vi "GetConnectorPaneTemplateForExecutionMode.vi"(8 "error in (no error)":errorcluster, 11 "execution mode":T2) -> (0 "error out":errorcluster, 3 "connector pane template":T1)   [LabVIEW 2015, in "VeriStandTestUtilities.lvlib"]
uses:
  VeriStandTestUtilities.lvlib
  <vilib>/NI Veristand/Custom Device API/Custom Device Execution Mode.ctl
  ConnectorPaneTemplate.ctl
  <userlib>/_OpenG.lib/file/file.llb/Build Path - Traditional - path__ogtk.vi
  <vilib>/NI Veristand/Custom Device API/Custom Device API.lvlib
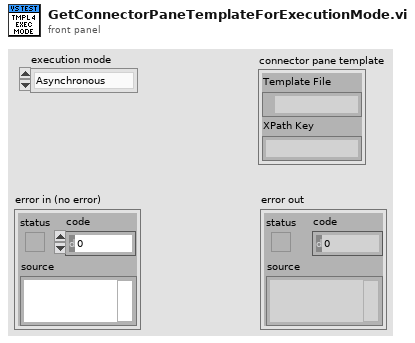
[diagram p1: front panel]
types:
  T1 = typedef "VeriStandTestUtilities.lvlib/ConnectorPaneTemplate.ctl" = cluster{"Template File":path, "XPath Key":string}
  T2 = typedef "Custom Device API.lvlib/Custom Device Execution Mode.ctl" = enum16{"Asynchronous", "Inline HW Interface", "Inline Model Interface", "Inline Timing and Sync", "Asynchronous Timing and Sync"}
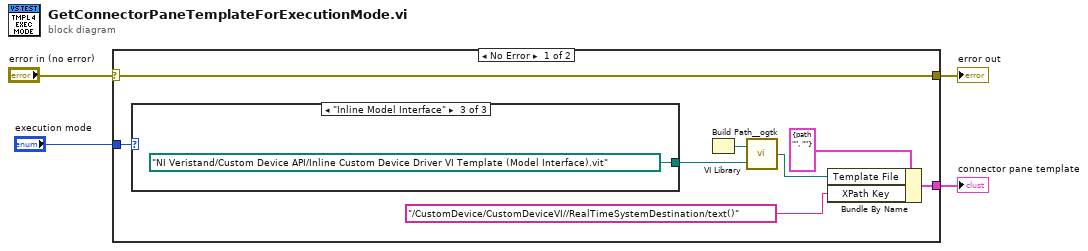
[diagram p0: block diagram]
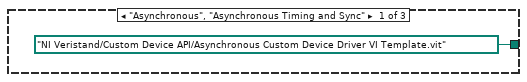
[diagram p2: hidden frame]
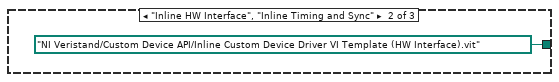
[diagram p3: hidden frame]
diagram:
  n1 = case shown="No Error" "error in (no error)" {
    selector: "error in (no error)" -> [w6 w16]
    tunnel: [w6 w16] -> w4
    tunnel: "execution mode" -> [w7 _]
    tunnel: [w5 _] -> w1
    frame No Error {
      n2 = case shown="\"Inline Model Interface\"" w7 {
        tunnel: [path "NI Veristand/Custom Device API/Asynchronous Custom Device Driver VI Template.vit" ("Folder Path") path "NI Veristand/Custom Device API/Inline Custom Device Driver VI Template (HW Interface).vit" ("Folder Path") path "NI Veristand/Custom Device API/Inline Custom Device Driver VI Template (Model Interface).vit" ("Folder Path")] -> w11
        frame "Asynchronous", "Asynchronous Timing and Sync" {
        }
        frame "Inline HW Interface", "Inline Timing and Sync" {
        }
        frame "Inline Model Interface" {
        }
      }
      n3 = VI Library() -> (path=w10:path)
      n4 = call-poly <userlib>:"Build Path__ogtk.vi"("name or relative path"=w11, "base path"=w10) -> ("appended path"=w12:path)
      n5 = Bundle By Name(cluster=T1 {"Template File"=path "", "XPath Key"=""} ("connector pane template 2"), "Template File"=w12, "XPath Key"="/CustomDevice/CustomDeviceVI//RealTimeSystemDestination/text()") -> (w5:T1)
    }
    frame Error {
    }
  }
  "error out" <- w4
  "connector pane template" <- w1
